vi "Add Error.vi"(5 "Error":errorcluster, 7 "Action":T1, 11 "Error list":errorcluster[](array[cluster])) -> (3 "Error list Out":errorcluster[](array[cluster]))   [LabVIEW 2017, in "VisionSystem.lvlib"]
uses:
  VisionSystem.lvlib
  ENUM_HW_Action.ctl
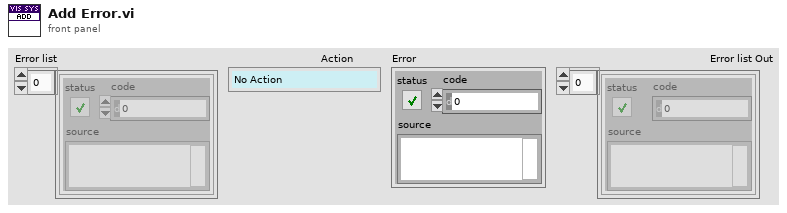
[diagram p1: front panel]
types:
  T1 = typedef "VisionSystem.lvlib/ENUM_HW_Action.ctl" = enum16{"No Action", "Reset Time", "Open Cam 0", "Open Cam 1", "Stop Camera", "Start Camera", "Acquire Camera", "Close Camera", "Read Avalable Cams", "Save Settings to File", "Restore Settings from File", "Open Image", "Close Image", "Set  Camera", "Read Cam Settings"}
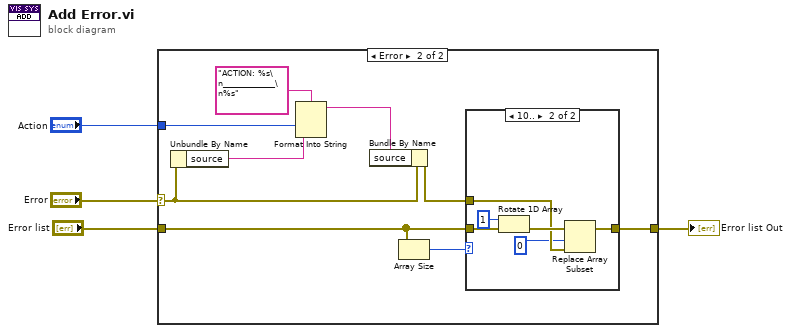
[diagram p0: block diagram]
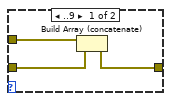
[diagram p3: hidden frame]
diagram:
  n1 = case shown="Error" "Error" {
    selector: "Error" -> [_ w14]
    tunnel: "Action" -> [_ w11]
    tunnel: "Error list" -> [w5 w7]
    tunnel: [w5 w12] -> w1
    frame No Error {
    }
    frame Error {
      n2 = Unbundle By Name(w14) -> ("source"=w9:string)
      n3 = Format Into String(format string="ACTION: %s\n_____________\n%s", w11, w9) -> (resulting string=w8:string)  [unwired: 2 in, 1 out]
      n4 = Bundle By Name(cluster=w14, "source"=w8) -> (w13:errorcluster)
      n5 = Array Size(array=w7) -> (size(s)=w6:i32)
      n6 = case shown="10.." w6 {
        tunnel: w13 -> [w17 w19]
        tunnel: [w16 w20] -> w12
        tunnel: w7 -> [w15 w23]
        frame ..9 {
          n7 = Build Array (concatenate)(w17, w15) -> (w16:errorcluster[])
        }
        frame 10.. {
          n8 = Rotate 1D Array(1:w23, 2:1 ("n")) -> (0:w21:errorcluster[])
          n9 = Replace Array Subset(array=w21, new element=w19, index=0) -> (w20:errorcluster[])
        }
      }
    }
  }
  "Error list Out" <- w1
